vi "sub_ui-property.vi"(7 "cmd":T1=enum."테스트정지") -> ()   [LabVIEW 2019]
uses:
  cmd_ui.ctl
  _ctrl/rw.ctl
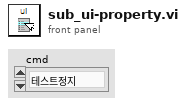
[diagram p1: front panel]
types:
  T1 = typedef "cmd_ui.ctl" = enum16{"초기화", "테스트시작", "테스트정지", "테스트종료"}
  T2 = typedef "rw.ctl" = enum16{"read", "write"}
  T3 = enum8{"Enabled", "Disabled", "Disabled and Grayed Out"}
  T4 = cluster{"시작":refnum<vi>, "RESET":refnum<vi>, "정지":refnum<vi>, "Exit":refnum<vi>, "대기":refnum<vi>, "Main":refnum<vi>, "시험세팅":refnum<vi>, "그래프":refnum<vi>}
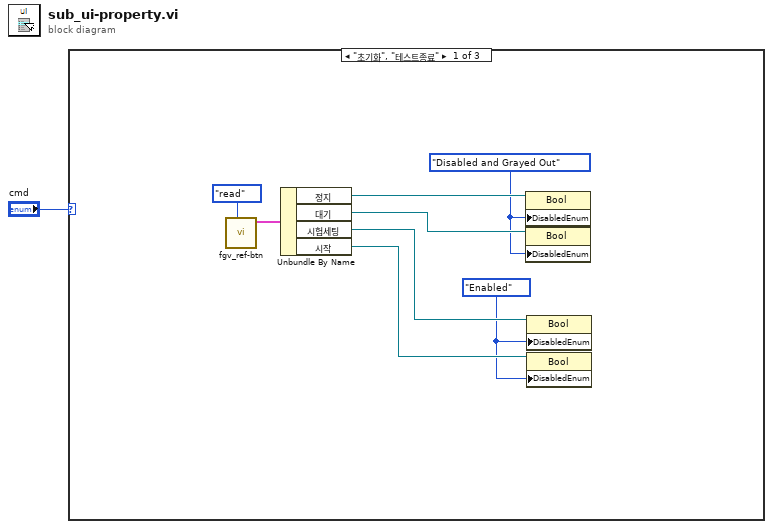
[diagram p0: block diagram]
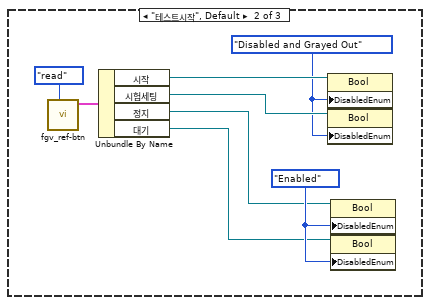
[diagram p2: hidden frame]
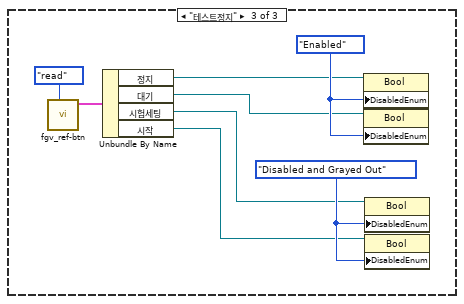
[diagram p3: hidden frame]
diagram:
  n1 = case shown="\"초기화\", \"테스트종료\"" "cmd" {
    frame "초기화", "테스트종료" {
      w2 = T3."Enabled" ("비활성화")
      w6 = T3."Disabled and Grayed Out" ("비활성화")
      n2 = call "fgv_ref-btn.vi"("cmd"=rw."read") -> ("ref 2"=w9:T4)  [unwired: 10 in]
      n3 = Unbundle By Name(w9) -> ("정지"=w8:refnum<vi>, "대기"=w7:refnum<vi>, "시험세팅"=w4:refnum<vi>, "시작"=w3:refnum<vi>)
      n4 = property class="Bool"(reference=w8, "DisabledEnum"=w6) -> ()  [unwired: 1 in, 2 out]
      n5 = property class="Bool"(reference=w7, "DisabledEnum"=w6) -> ()  [unwired: 1 in, 2 out]
      n6 = property class="Bool"(reference=w4, "DisabledEnum"=w2) -> ()  [unwired: 1 in, 2 out]
      n7 = property class="Bool"(reference=w3, "DisabledEnum"=w2) -> ()  [unwired: 1 in, 2 out]
    }
    frame "테스트시작", Default {
      w12 = T3."Enabled" ("비활성화")
      w14 = T3."Disabled and Grayed Out" ("비활성화")
      n8 = call "fgv_ref-btn.vi"("cmd"=rw."read") -> ("ref 2"=w17:T4)  [unwired: 10 in]
      n9 = Unbundle By Name(w17) -> ("시작"=w16:refnum<vi>, "시험세팅"=w15:refnum<vi>, "정지"=w11:refnum<vi>, "대기"=w10:refnum<vi>)
      n10 = property class="Bool"(reference=w16, "DisabledEnum"=w14) -> ()  [unwired: 1 in, 2 out]
      n11 = property class="Bool"(reference=w15, "DisabledEnum"=w14) -> ()  [unwired: 1 in, 2 out]
      n12 = property class="Bool"(reference=w11, "DisabledEnum"=w12) -> ()  [unwired: 1 in, 2 out]
      n13 = property class="Bool"(reference=w10, "DisabledEnum"=w12) -> ()  [unwired: 1 in, 2 out]
    }
    frame "테스트정지" {
      w25 = T3."Disabled and Grayed Out" ("비활성화")
      w21 = T3."Enabled" ("비활성화")
      n14 = call "fgv_ref-btn.vi"("cmd"=rw."read") -> ("ref 2"=w18:T4)  [unwired: 10 in]
      n15 = Unbundle By Name(w18) -> ("정지"=w19:refnum<vi>, "대기"=w20:refnum<vi>, "시험세팅"=w23:refnum<vi>, "시작"=w24:refnum<vi>)
      n16 = property class="Bool"(reference=w19, "DisabledEnum"=w21) -> ()  [unwired: 1 in, 2 out]
      n17 = property class="Bool"(reference=w20, "DisabledEnum"=w21) -> ()  [unwired: 1 in, 2 out]
      n18 = property class="Bool"(reference=w23, "DisabledEnum"=w25) -> ()  [unwired: 1 in, 2 out]
      n19 = property class="Bool"(reference=w24, "DisabledEnum"=w25) -> ()  [unwired: 1 in, 2 out]
    }
  }
